vi "Write Data.vi"(8 "error in (no error)":errorcluster, 9 "Data":variant, 10 "LogicName":string, 11 "PLC_Module in":refnum<class "PLC_Module.lvclass">) -> (0 "error out":errorcluster, 3 "PLC_Module out":refnum<class "PLC_Module.lvclass">)   [LabVIEW 2025, in "PLC_Module.lvlib" / "PLC_Module.lvclass"]
uses:
  PLC_Module.lvclass
  PLC_Module.lvclass/PLC_Module.ctl
  PLC_Abstr/PLC_Abstr Messages/Write Data Msg/Write Data Msg.lvclass
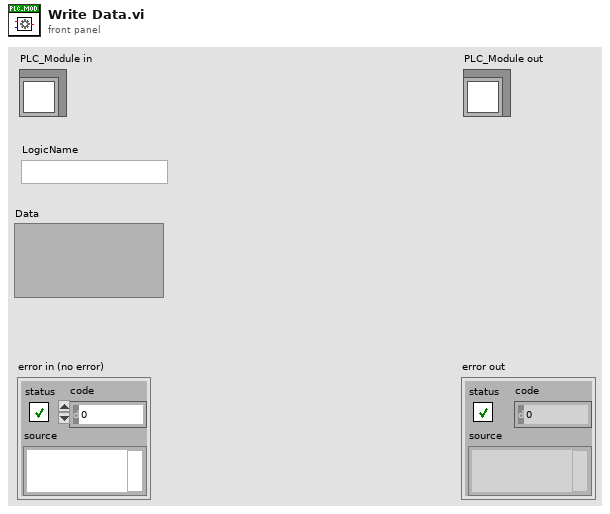
[diagram p1: front panel]
types:
  T1 = typedef "PLC_Module.lvlib/PLC_Module.lvclass/PLC_Data_Config.ctl" = map{string, cluster{"Config":T2, "Value":string}}
  T2 = typedef "PLC_Module.lvlib/PLC_Module.lvclass/PLC_Data.ctl" = cluster{"StartAddress":u32, "Direction":enum16{"PC->PLC", "PLC->PC"}, "DataType":T3, "DefaultValue":string, "Description":string}
  T3 = typedef "PLC_Module.lvlib/PLC_Module.lvclass/PLC_Data_Type.ctl" = enum16{"U8", "U32", "U32_Array", "String"}
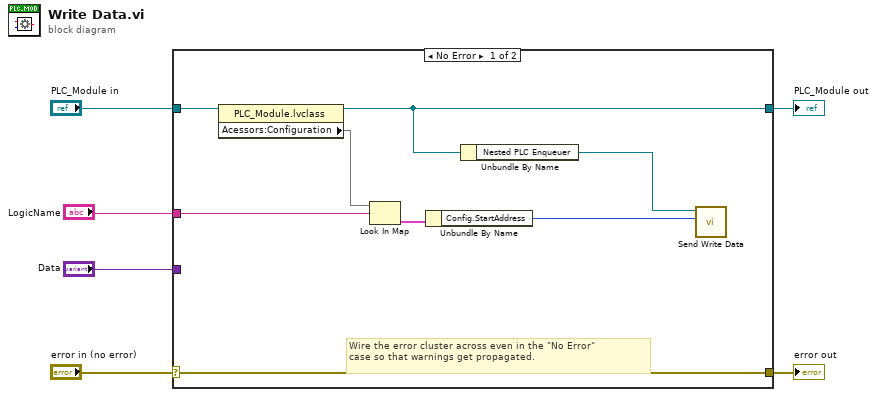
[diagram p0: block diagram]
diagram:
  n1 = case shown="No Error" "error in (no error)" {
    selector: "error in (no error)" -> [w13 w16]
    tunnel: [w13 w16] -> w5
    tunnel: [w10 w15] -> w3
    tunnel: "PLC_Module in" -> [w14 w15]
    tunnel: "LogicName" -> [w11 _]
    tunnel: "Data" -> [_ _]
    frame No Error {
      # "Wire the error cluster across even in the \"No Error\"\ncase so that warnings get propagated."
      n2 = property class="PLC_Module.lvclass"(reference=w14) -> (reference out=w10:refnum<class "PLC_Module.lvclass">, "Acessors:Configuration"=w12:T1)  [unwired: 1 in, 1 out]
      n3 = Look In Map(map=w12, key=w11) -> (value=w8:cluster{"Config":T2, "Value":string})  [unwired: 1 in, 1 out]
      n4 = Unbundle By Name(w8) -> ("Config.StartAddress"=w7:u32)
      n5 = Unbundle By Name(w10) -> ("Nested PLC Enqueuer"=w9:refnum<class "Message Enqueuer.lvclass">)
      n6 = call "Send Write Data.vi"("Start Address"=w7, "Message Enqueuer"=w9) -> ()  [unwired: 8 in, 2 out]
    }
    frame Error {
    }
  }
  "error out" <- w5
  "PLC_Module out" <- w3
